vi "Format Table Cells into Table Row.vi"(11 "Table Cells":string[](array[string])) -> (3 "Table Row Text":string)   [LabVIEW 2023, in "Confluence Formatting.lvlib"]
uses:
  Confluence Formatting.lvlib
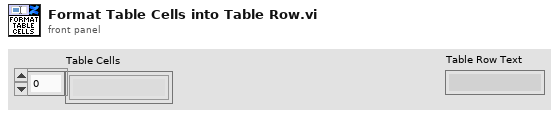
[diagram p1: front panel]
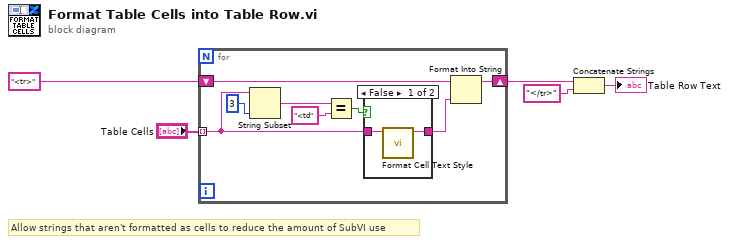
[diagram p0: block diagram]
diagram:
  # "Allow strings that aren't formatted as cells to reduce the amount of SubVI use"
  n1 = for {
    tunnel: "Table Cells" -> [w8] mode=indexing
    shift-right: [w12] -> w3
    shift-left: "<tr>" -> [w13]
    n2 = String Subset(string=w8, length (rest)=3 ("length (rest)")) -> (substring=w10:string)  [unwired: 1 in]
    n3 = Equal?(x=w10, y="<td") -> (x = y?=w6:bool)
    n4 = case shown="False" w6 {
      tunnel: w8 -> [w15 w16]
      tunnel: [w14 w16] -> w7
      frame False {
        n5 = call "Format Cell Text Style.vi"("String"=w15) -> ("Formatted Text"=w14:string)  [unwired: 9 in, 1 out]
      }
      frame True {
      }
    }
    n6 = Format Into String(initial string=w13, w7) -> (resulting string=w12:string)  [unwired: 2 in, 1 out]
  }
  n7 = Concatenate Strings(w3, "</tr>" ("string")) -> (→"Table Row Text":string)
